vi "Configure List.vi"   [LabVIEW 2020, in "TDK-Lambda Z.lvlib"]
uses:
  TDK-Lambda Z.lvlib
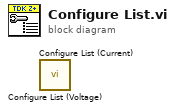
[diagram p0: block diagram]
diagram:
  n1 = call "Configure List (Voltage).vi"() -> ()  [unwired: 10 in, 2 out]
  n2 = call "Configure List (Current).vi"() -> ()  [unwired: 10 in, 2 out]
